vi "GetFSS_InnerTunnelTerminals.vi"(5 "Tunnel in":refnum<class "FlatSequenceInnerTunnel.lvclass">, 6 "error in":errorcluster, 9 "VI Interpreter in":refnum<class "VI Interpreter.lvclass">) -> (0 "error out":errorcluster, 3 "VI Interpreter out":refnum<class "VI Interpreter.lvclass">, 4 "Tunnel out":refnum<class "FlatSequenceInnerTunnel.lvclass">)   [LabVIEW 2014, in "Raspberry Pi Compatible Compiler for LabVIEW.lvlib" / "VI Interpreter.lvclass"]
uses:
  VI Interpreter.lvclass
  FlatSequenceInnerTunnel/FlatSequenceInnerTunnel.lvclass
  FlatSequenceInnerTunnel/FlatSequenceInnerTunnel.lvclass/FlatSequenceInnerTunnel.ctl
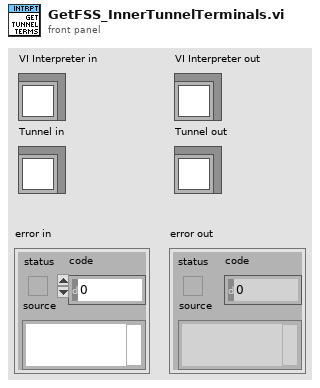
[diagram p1: front panel]
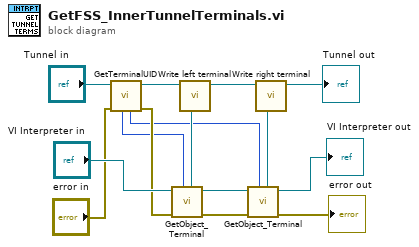
[diagram p0: block diagram]
diagram:
  n1 = call "GetTerminalUID.vi"("error in"="error in", "Tunnel in"="Tunnel in") -> ("error out"=w3:errorcluster, "Tunnel out"=w7:refnum<class "FlatSequenceInnerTunnel.lvclass">, "right terminal UID"=w1:i32, "left terminal UID"=w2:i32)  [unwired: 4 in]
  n2 = call "GetObject_Terminal.vi"("UID"=w2, "error in"=w3, "VI Interpreter in"="VI Interpreter in") -> ("error out"=w8:errorcluster, "VI Interpreter out"=w10:refnum<class "VI Interpreter.lvclass">, "Terminal"=w5:refnum<class "Terminal.lvclass">)  [unwired: 3 in, 1 out]
  n3 = call "Write left terminal.vi"("left terminal"=w5, "FlatSequenceInnerTunnel in"=w7) -> ("FlatSequenceInnerTunnel out"=w6:refnum<class "FlatSequenceInnerTunnel.lvclass">)  [unwired: 7 in]
  n4 = call "GetObject_Terminal.vi"("UID"=w1, "error in"=w8, "VI Interpreter in"=w10) -> ("error out"=→"error out":errorcluster, "VI Interpreter out"=→"VI Interpreter out":refnum<class "VI Interpreter.lvclass">, "Terminal"=w12:refnum<class "Terminal.lvclass">)  [unwired: 3 in, 1 out]
  n5 = call "Write right terminal.vi"("right terminal"=w12, "FlatSequenceInnerTunnel in"=w6) -> ("FlatSequenceInnerTunnel out"=→"Tunnel out":refnum<class "FlatSequenceInnerTunnel.lvclass">)  [unwired: 7 in]
